vi "Pose2d_RelativeTo.vi"(9 "other POSE":T1 {"ROTATION"."SIN" format="%13.4f"; "ROTATION"."COS" format="%13.4f"; "ROTATION"."VALUE" format="%13.4f"; "TRANSLATION"."Y" format="%14.3f"; "TRANSLATION"."X" format="%14.3f"}, 11 "in POSE":T1 {"ROTATION"."SIN" format="%13.4f"; "ROTATION"."COS" format="%13.4f"; "ROTATION"."VALUE" format="%13.4f"; "TRANSLATION"."Y" format="%14.3f"; "TRANSLATION"."X" format="%14.3f"}) -> (3 "out POSE":T1 {"ROTATION"."SIN" format="%13.4f"; "ROTATION"."COS" format="%13.4f"; "ROTATION"."VALUE" format="%13.4f"; "TRANSLATION"."Y" format="%14.3f"; "TRANSLATION"."X" format="%14.3f"})   [LabVIEW 2019, in "Trajectory_Library.lvlib"]
doc: "Returns the other pose relative to the current pose.\n\nThis function can often be used for trajectory tracking or pose stabilization algorithms to get the error between the reference and the current pose.\n\nParameters:\n - IN POSE - The POSE data structure\n - OTHER POSE - The pose that is the origin of the new coordinate frame that the current pose will be converted into.\n\nReturn:\n - OUT POSE - The current pose relative to the new origin pose."
uses:
  Trajectory_Library.lvlib
  TypeDef/POSE2D.ctl
  TypeDef/TRANSLATION2D.ctl
  TypeDef/ROTATION2D.ctl
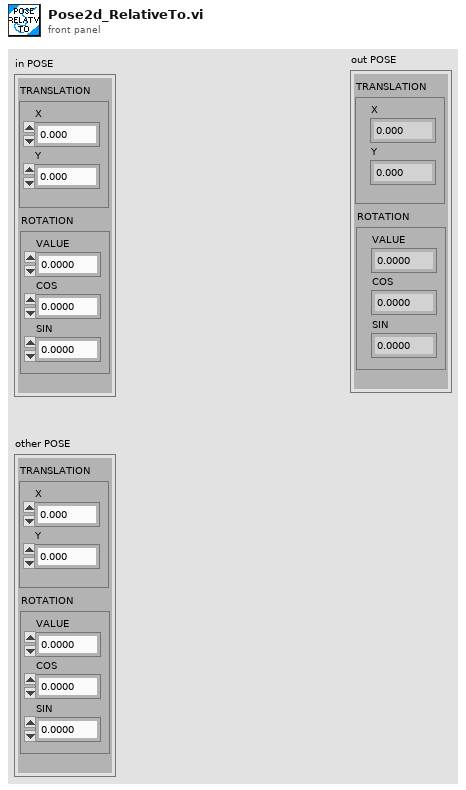
[diagram p1: front panel]
types:
  T1 = typedef "Trajectory_Library.lvlib/POSE2D.ctl" = cluster{"TRANSLATION":T2, "ROTATION":T3}
  T2 = typedef "Trajectory_Library.lvlib/TRANSLATION2D.ctl" = cluster{"X":dbl, "Y":dbl}
  T3 = typedef "Trajectory_Library.lvlib/ROTATION2D.ctl" = cluster{"VALUE":dbl, "COS":dbl, "SIN":dbl}
  T4 = typedef "Trajectory_Library.lvlib/TRANSFORM2D.ctl" = cluster{"TRANSLATION":T2, "ROTATION":T3, "xF":bool}
  T5 = typedef "WPILib_Math.lvlib/POSE2D.ctl" = cluster{"TRANSLATION":T6, "ROTATION":T7}
  T6 = typedef "WPILib_Math.lvlib/TRANSLATION2D.ctl" = cluster{"X":dbl, "Y":dbl}
  T7 = typedef "WPILib_Math.lvlib/ROTATION2D.ctl" = cluster{"VALUE":dbl, "COS":dbl, "SIN":dbl}
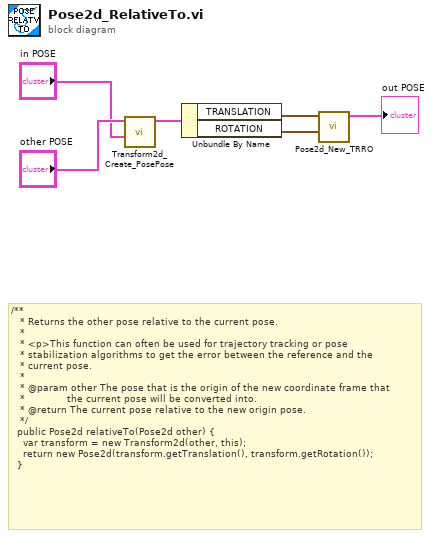
[diagram p0: block diagram]
diagram:
  # "/**\n   * Returns the other pose relative to the current pose.\n   *\n   * <p>This function can often be used for trajectory tracking or pose\n   * stabilization algorithms to get the error between the reference and the\n   * current pose.\n   *\n   * @param other The pose that is the origin of the new coordinate frame that\n   *              the current pose will be converted into.\n   * @return The current pose relative to the new origin pose.\n   */\n  public Pose2d relativeTo(Pose2d other) {\n    var transform = new Transform2d(other, this);\n    return new Pose2d(transform.getTranslation(), transform.getRotation());\n  }"
  n1 = call "Transform2d_Create_PosePose.vi"("last POSE"="in POSE", "initial POSE"="other POSE") -> ("TRANSFORM"=w6:T4)  [unwired: 9 in]
  n2 = Unbundle By Name(w6) -> ("TRANSLATION"=w2:T2, "ROTATION"=w1:T3)
  n3 = call "Pose2d_New_TRRO.vi"("ROTATION"=w1, "TRANSLATION"=w2) -> ("outPOSE"=→"out POSE":T5)  [unwired: 9 in]
